vi "FileTo2dArray.vi"(1 "file path (dialog if empty)":path) -> (0 "Array":string[][](array[string]))   [LabVIEW 2014, in "Panels.lvlib"]
uses:
  Panels.lvlib
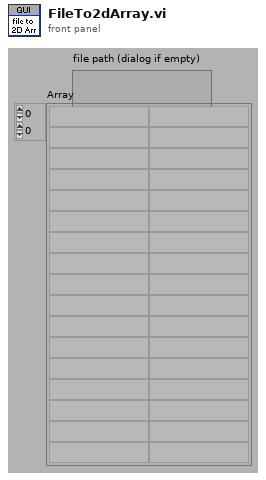
[diagram p1: front panel]
types:
  T1 = enum16{"open", "replace", "create", "open or create", "replace or create", "replace or create with confirmation"}
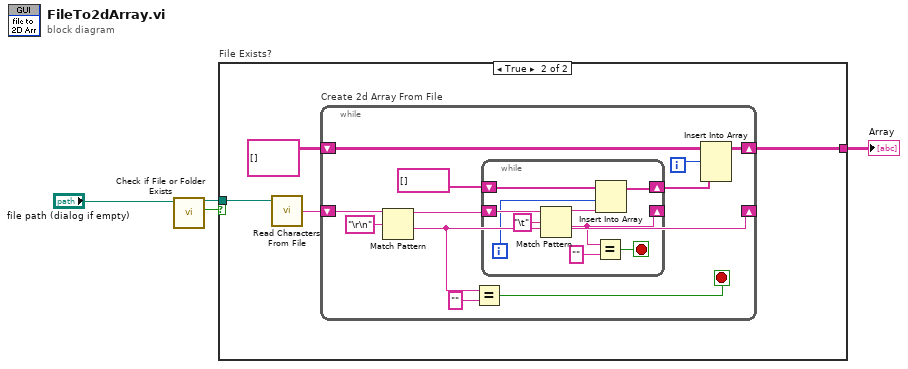
[diagram p0: block diagram]
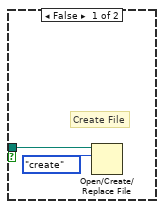
[diagram p2: hidden frame]
diagram:
  n1 = call <vilib>:"Check if File or Folder Exists.vi"("path"="file path (dialog if empty)") -> ("file or folder exists?"=w2:bool, "dup path"=w3:path)  [unwired: 8 in, 1 out]
  n2 = case "File Exists?" shown="True" w2 {
    tunnel: w3 -> [w6 w8]
    tunnel: [_ w7] -> w1
    frame False {
      # "Create File"
      n3 = Open/Create/Replace File(file path (use dialog)=w6, operation (0:open)=T1."create") -> ()  [unwired: 4 in, 3 out]
    }
    frame True {
      n4 = call <vilib>:"Read Characters From File.vi"("file path (dialog if empty)"=w8) -> ("character string"=w10:string)  [unwired: 5 in, 3 out]
      n5 = while "Create 2d Array From File" {
        shift-right: [w18] -> _
        shift-left: w10 -> [w21]
        shift-right: [w14] -> w7
        shift-left: string[][] [] -> [w13]
        i -> [w11]
        stop <- w16 stop-if-true
        n6 = Match Pattern(string=w21, regular expression="\r\n") -> (before substring=w19:string, after substring=w18:string)  [unwired: 1 in, 2 out]
        n7 = Equal?(x=w18, y="") -> (x = y?=w16:bool)
        n8 = while {
          shift-right: [w24] -> _
          shift-left: w19 -> [w30]
          shift-right: [w25] -> w12
          shift-left: string[] [] -> [w28]
          i -> [w26]
          stop <- w22 stop-if-true
          n9 = Match Pattern(string=w30, regular expression="\t") -> (before substring=w27:string, after substring=w24:string)  [unwired: 1 in, 2 out]
          n10 = Equal?(x=w24, y="") -> (x = y?=w22:bool)
          n11 = Insert Into Array(array=w28, index=w26, new element=w27) -> (w25:string[])
        }
        n12 = Insert Into Array(array=w13, index (row)=w11, new element=w12) -> (w14:string[][])  [unwired: 1 in]
      }
    }
  }
  "Array" <- w1
